vi "ASAP_SubVI_rt.vi"(6 "Reset":bool, 7 "Micron config":T1, 8 "error in":errorcluster, 9 "Configuration":T4, 10 "Time in":cluster{"t0":timestamp, "dt":dbl}, 11 "ADC data in":sgl[][](array[numeric])=[[0.4233891, 0.059737563, -0.3452632, -0.43708423, -0.1850327, 0.11627349, 0.3480983, 0.14520556, -0.018593404, -0.042756785, 0.0034736844, 0.02845318, -0.059975192, -0.3118025, -0.19130558, 0.09030185, 0.36043605], [0.6090162, 0.02373252, -0.52186435, -0.6243751, -0.2834785, 0.15024628, 0.48947865, 0.24355544, 0.052680574, 0.005137917, -0.03373152, -0.046069246, -0.18644089, -0.46828866, -0.19741842, 0.22753717, 0.5495514], [-0.36270568, 0.031333584, 0.3305598, 0.36922133, 0.17977042, -0.0914356, -0.29096755, -0.16731821, -0.07733762, -0.032019284, 0.04986418, 0.07868422, 0.16904892, 0.2834651, 0.064586245, -0.19497009, -0.3473115], [-0.6450181, 0.10571201, 0.61151254, 0.6368443, 0.17301747, -0.31877947, -0.51290303, -0.13209727, 0.06778669, 0.057593264, -0.031955272, -0.06567199, 0.19175611, 0.49285513, 0.23913881, -0.27019665, -0.6145497], [0.46957177, -0.13065708, -0.48157057, -0.46508822, -0.10884603, 0.27197546, 0.37166968, 0.08025244, -0.055926625, -0.03766807, 0.027317023, 0.049336106, -0.17896785, -0.37037078, -0.16486987, 0.23949087, 0.4787091], [0.6681609, -0.26571602, -0.7523299, -0.68411183, -0.18660091, 0.41935652, 0.55092764, 0.16146386, -0.011424401, -0.025378352, -0.01148841, -0.0049274913, -0.35867313, -0.5398829, -0.15688474, 0.44660845, 0.748461], [-0.3118825, 0.18517919, 0.40708274, 0.34915444, 0.12969938, -0.21727721, -0.29184768, -0.13747403, -0.0707447, -0.0026391712, 0.06805873, 0.0856772, 0.2530928, 0.25218067, -0.009680157, -0.29677638, -0.40475965], [-0.6122774, 0.44387203, 0.8820655, 0.6474379, 0.013395073, -0.6203265, -0.51136684, -0.011152362, 0.15547901, 0.035622187, -0.099948786, -0.11585501, 0.43435067, 0.58534867, 0.18177071, -0.5484282, -0.8615302], [-0.06624807, -0.05802292, -0.042420737, -0.031315185, -0.031459205, -0.04258076, -0.05151001, -0.051558014, -0.04872562, -0.048101533, -0.049829774, -0.051766045, -0.044020962, -0.033891544, -0.031091152, -0.04093253, -0.05603864], [-0.022401936, -0.022561958, -0.02249795, -0.022241915, -0.022017883, -0.022001881, -0.022113897, -0.022161903, -0.022225913, -0.022241915, -0.022321925, -0.022481948, -0.02243394, -0.022225913, -0.021953873, -0.021873862, -0.022113897], [-0.044613045, -0.04464505, -0.04464505, -0.04464505, -0.044629045, -0.044629045, -0.044629045, -0.044613045, -0.044613045, -0.044629045, -0.04459704, -0.044613045, -0.04464505, -0.044565037, -0.044613045, -0.044565037, -0.04458104], [-0.044565037, -0.044565037, -0.044533033, -0.044533033, -0.044549033, -0.044565037, -0.044549033, -0.04459704, -0.04451703, -0.044533033, -0.044533033, -0.044565037, -0.04459704, -0.044629045, -0.044613045, -0.044613045, -0.044613045]]) -> (0 "error out":errorcluster, 2 "Time out":cluster{"t0":timestamp, "dt":dbl}, 3 "XYZ out":sgl[][](array[numeric]) format="%#.2f", 4 "Position valid":bool, 5 "No pose":bool)   [LabVIEW 2014]
uses:
  initialization/configuration.ctl
  initialization/asap_calibration.ctl
  <vilib>/Analysis/Matrix/Datatypes/RealMatrix.ctl
  micron/labview/initialization/micron_config.ctl
  micron/labview/manipulator/squiggle/Host/i2c_interface.ctl
  micron/labview/manipulator/squiggle/Host/fpga_reference.ctl
  micron/labview/testing/Micron params.ctl
  micron/labview/testing/stimulus.ctl
  micron/labview/testing/injection_point.ctl
  micron/labview/filtering/goal_loop_parms.ctl
  micron/labview/testing/mode_conrols.ctl
  micron/labview/testing/manipulator_cal.ctl
  testing/probe_calibration.ctl
  micron/labview/host/network_params.ctl
  micron/labview/cancellation/sq_control_params.ctl
  micron/labview/cancellation/decoupled_gain.ctl
  micron/labview/cancellation/estimation_controls.ctl
  <vilib>/Analysis/4window.llb/Hanning Window (DBL).vi
  <vilib>/Analysis/4window.llb/AllCosWindow (DBL).vi
  <vilib>/Analysis/NI_AALPro.lvlib
  <vilib>/Analysis/Matrix/NI_Matrix.lvlib
panel:
  in  "Impulse filter":bool=TRUE
  in  "Window":bool=TRUE
  # "Options:"
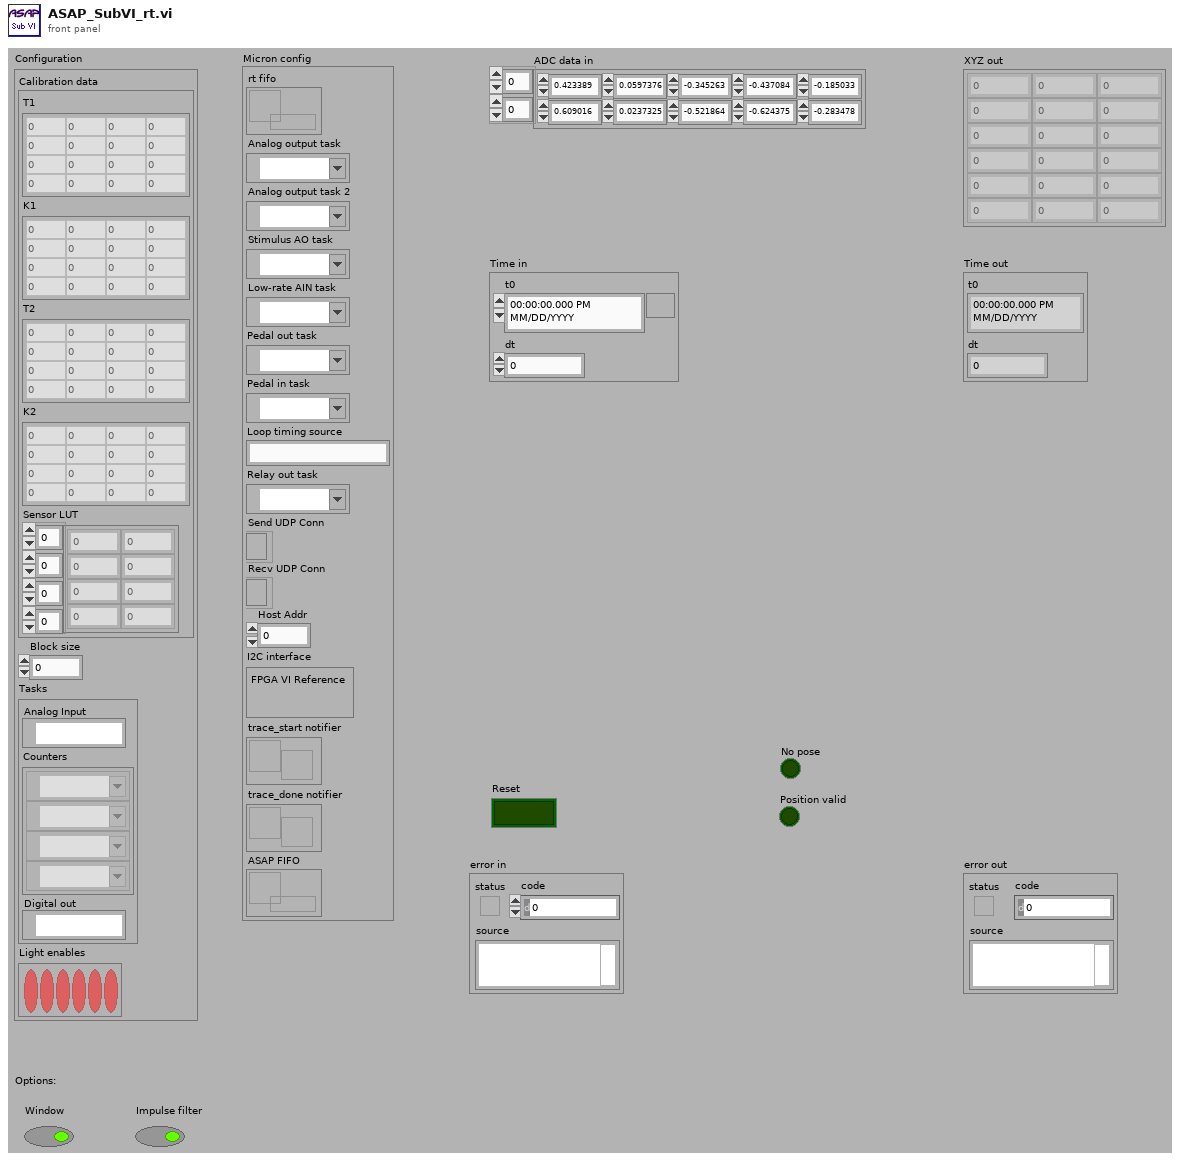
[diagram p1: front panel]
types:
  T1 = typedef "micron_config.ctl" = cluster{"rt fifo":refnum<k33>, "Analog output task":refnum<k21>, "Analog output task 2":refnum<k21>, "Stimulus AO task":refnum<k21>, "Low-rate AIN task":refnum<k21>, "Pedal out task":refnum<k21>, "Pedal in task":refnum<k21>, "Loop timing source":string, "Relay out task":refnum<k21>, "Send UDP Conn":refnum<k16>, "Recv UDP Conn":refnum<k16>, "Host Addr":u32, "I2C interface":T2, "trace_start notifier":refnum<notifier>, "trace_done notifier":refnum<notifier>, "ASAP FIFO":refnum<k33>}
  T2 = typedef "i2c_interface.ctl" = cluster{"FPGA VI Reference":T3}
  T3 = typedef "fpga_reference.ctl" = refnum<k20>
  T4 = typedef "configuration.ctl" = cluster{"Calibration data":T5, "Block size":i32, "Tasks":cluster{"Analog Input":refnum<k21>, "Counters":refnum<k21>[], "Digital out":refnum<k21>}, "Light enables":bool[]}
  T5 = typedef "asap_calibration.ctl" = cluster{"T1":T6, "K1":T6, "T2":T6, "K2":T6, "Sensor LUT":sgl[][][][]}
  T6 = typedef "NI_Matrix.lvlib/RealMatrix.ctl" = dbl[][]
  T7 = cluster{"Block size":i32, "Light enables":bool[], "Window":bool}
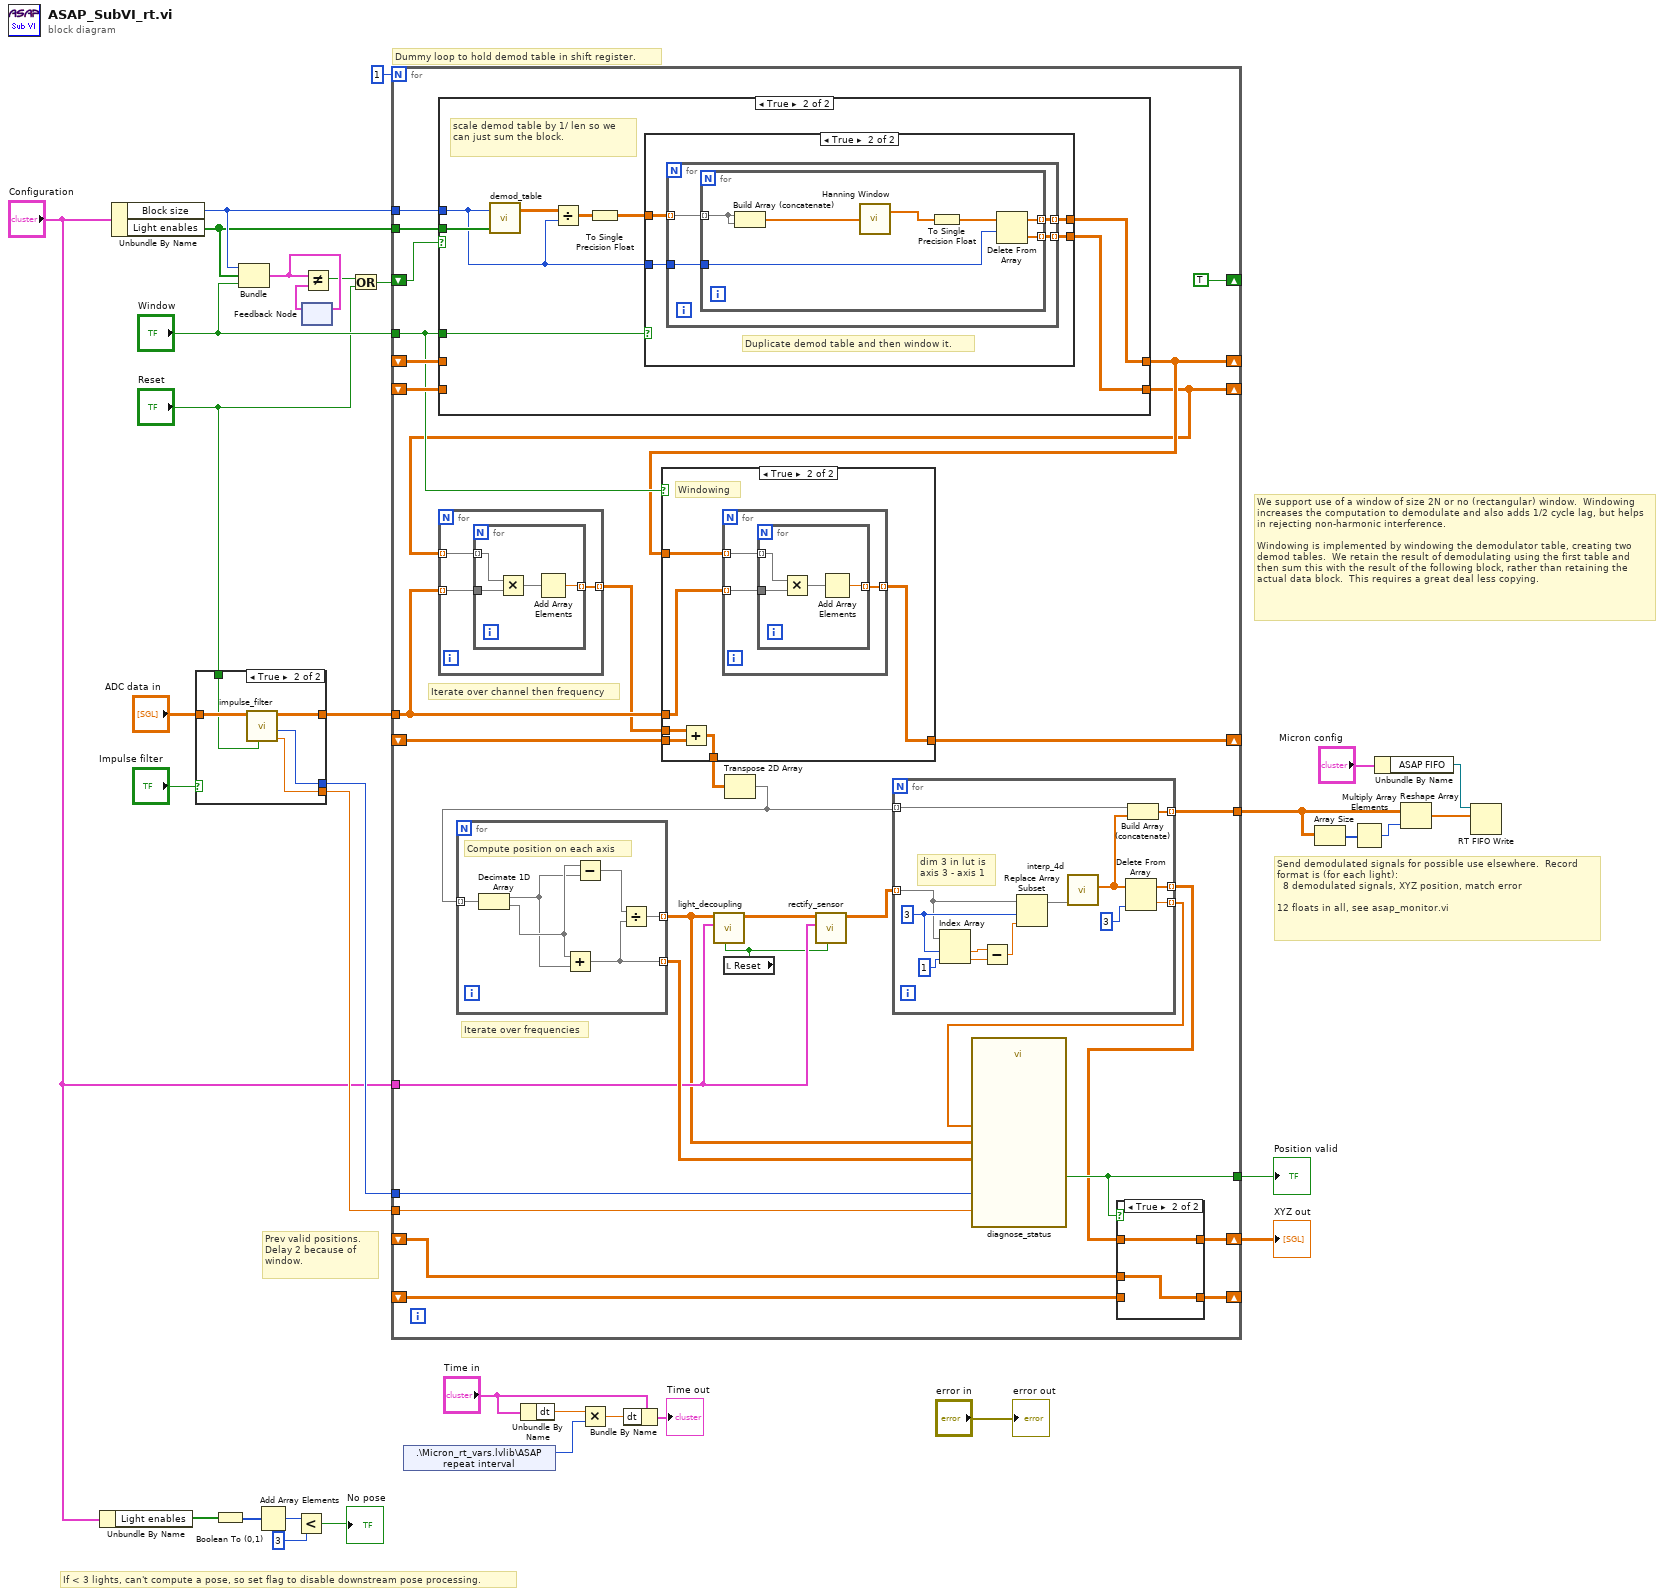
[diagram p0: block diagram]
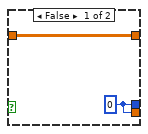
[diagram p2: hidden frame]
diagram:
  # "If < 3 lights, can't compute a pose, so set flag to disable downstream pose processing."
  # "Send demodulated signals for possible use elsewhere.  Record format is (for each light):\n  8 demodulated signals, XYZ position, match error\n\n12 floats in all, see asap_monitor.vi"
  # "Prev valid positions. Delay 2 because of window."
  # "We support use of a window of size 2N or no (rectangular) window.  Windowing increases the computation to demodulate and also adds 1/2 cycle lag, but helps in rejecting non-harmonic interference.\n\nWindowing is implemented by windowing the demodulator table, creating two demod tables.  We retain the result of demodulating using the first table and then sum this with the result of the following block, rather than retaining the actual data block.  This requires a great deal less copying."
  # "Dummy loop to hold demod table in shift register."
  n1 = Unbundle By Name("Configuration") -> ("Light enables"=w5:bool[])
  n2 = Unbundle By Name("Configuration") -> ("Block size"=w26:i32, "Light enables"=w25:bool[])
  n3 = case shown="True" "Impulse filter" {
    tunnel: "ADC data in" -> [w36 w39]
    tunnel: [w36 w38] -> w20
    tunnel: [w35 w41] -> w18
    tunnel: [w35 w40] -> w17
    tunnel: "Reset" -> [_ w37]
    frame False {
      w35 = 0 ("Repair count")
    }
    frame True {
      n4 = call "impulse_filter.vi"("Reset"=w37, "Signal in"=w39) -> ("RMS mismatch"=w40:sgl, "Repair count"=w41:i32, "Signal out"=w38:sgl[][])  [unwired: 7 in]
    }
  }
  n5 = Boolean To (0,1)(Boolean=w5) -> (0, 1=w4:i16[])
  n6 = Bundle("Block size"=w26, "Light enables"=w25, "Window"="Window") -> (w22:T7)  [unwired: 1 in]
  n7 = Add Array Elements(numeric array=w4) -> (sum=w3:i16)
  n8 = Less?(x=w3, y=i16 3) -> (x < y?=→"No pose":bool)
  n9 = feedback-in #1(w22) -> ()
  n10 = feedback #1() -> (w23:T7)  [unwired: 1 in]
  n11 = Not Equal?(x=w22, y=w23) -> (x != y?=w8:bool)
  n12 = Or(x=w8, y="Reset") -> (x .or. y?=w9:bool)
  n13 = for {
    N: 1 -> [_]
    tunnel: w20 -> [w64]
    shift-right: [w60] -> _
    shift-left: _ -> [w70]
    shift-right: [TRUE] -> _
    shift-left: w9 -> [w72]
    tunnel: w26 -> [w69]
    tunnel: w25 -> [w67]
    tunnel: [w51] -> w11
    shift-right: [w57] -> w28
    shift-left: _ -> [w56]
    tunnel: "Window" -> [w65]
    shift-right: [w59] -> _
    shift-left: _ -> [w66]
    shift-right: [w62] -> _
    shift-left: _ -> [w61]
    tunnel: [w46] -> w12
    shift-right: [w55] -> _
    shift-left: _ -> [w54]
    tunnel: w18 -> [w53]
    tunnel: w17 -> [w52]
    tunnel: "Configuration" -> [w45]
    # "Iterate over channel then frequency"
    # "Iterate over frequencies"
    n14 = case shown="True" w72 {
      tunnel: [w105 w107] -> w60
      tunnel: w70 -> [w105 _]
      tunnel: w69 -> [_ w108]
      tunnel: w67 -> [_ w111]
      tunnel: w65 -> [_ w110]
      tunnel: [w104 w106] -> w59
      tunnel: w66 -> [w104 _]
      frame False {
      }
      frame True {
        # "scale demod table by 1/ len so we can just sum the block."
        n15 = call "demod_table.vi"("Light enables"=w111, "Block size"=w108) -> ("Sine table"=w113:dbl[][][])  [unwired: 1 out]
        n16 = Divide(x=w113, y=w108) -> (x/y=w112:dbl[][][])
        n17 = To Single Precision Float(number=w112) -> (single precision float=w109:sgl[][][])
        n18 = case shown="True" w110 {
          tunnel: w109 -> [w114 w115]
          tunnel: w108 -> [_ w118]
          tunnel: [w114 w117] -> w107
          tunnel: [w114 w116] -> w106
          frame False {
          }
          frame True {
            # "Duplicate demod table and then window it."
            n19 = for {
              tunnel: w115 -> [w122] mode=indexing
              tunnel: [w121] -> w117 mode=indexing
              tunnel: [w120] -> w116 mode=indexing
              tunnel: w118 -> [w119]
              n20 = for {
                tunnel: w122 -> [w125] mode=indexing
                tunnel: [w129] -> w121 mode=indexing
                tunnel: [w128] -> w120 mode=indexing
                tunnel: w119 -> [w127]
                n21 = Build Array (concatenate)(w125, w125) -> (w123:sgl[])
                n22 = call-poly <vilib>:"Hanning Window.vi"("X"=w123) -> ("Windowed X"=w124:dbl[])  [unwired: 1 out]
                n23 = To Single Precision Float(number=w124) -> (single precision float=w126:sgl[])
                n24 = Delete From Array(array=w126, length=w127) -> (deleted portion=w128:sgl[], array with subset deleted=w129:sgl[])  [unwired: 1 in]
              }
            }
          }
        }
      }
    }
    n25 = for {
      tunnel: w64 -> [w132] mode=indexing
      tunnel: [w131] -> w63 mode=indexing
      tunnel: w59 -> [w130] mode=indexing
      n26 = for {
        tunnel: w132 -> [w136]
        tunnel: [w134] -> w131 mode=indexing
        tunnel: w130 -> [w133] mode=indexing
        n27 = Multiply(x=w133, y=w136) -> (x*y=w135:sgl[])
        n28 = Add Array Elements(numeric array=w135) -> (sum=w134:sgl)
      }
    }
    n29 = case shown="True" w65 {
      tunnel: w60 -> [_ w96]
      tunnel: w64 -> [_ w95]
      tunnel: w63 -> [w89 w94]
      tunnel: [w89 w93] -> w58
      tunnel: [w90 w92] -> w62
      tunnel: w61 -> [w90 w91]
      frame False {
        # "Not windowing"
      }
      frame True {
        # "Windowing"
        n30 = Add(x=w94, y=w91) -> (x+y=w93:sgl[][])
        n31 = for {
          tunnel: w95 -> [w99] mode=indexing
          tunnel: [w98] -> w92 mode=indexing
          tunnel: w96 -> [w97] mode=indexing
          n32 = for {
            tunnel: w99 -> [w103]
            tunnel: [w101] -> w98 mode=indexing
            tunnel: w97 -> [w100] mode=indexing
            n33 = Multiply(x=w100, y=w103) -> (x*y=w102:sgl[])
            n34 = Add Array Elements(numeric array=w102) -> (sum=w101:sgl)
          }
        }
      }
    }
    n35 = local read "Reset"() -> (w44:bool)
    n36 = Transpose 2D Array(2D array=w58) -> (transposed array=w47:sgl[][])
    n37 = for {
      tunnel: w47 -> [w142] mode=indexing
      tunnel: [w140] -> w68 mode=indexing
      tunnel: [w137] -> w42 mode=indexing
      # "Compute position on each axis"
      n38 = Decimate 1D Array(w142) -> (w139:sgl[], w141:sgl[])
      n39 = Add(x=w141, y=w139) -> (x+y=w140:sgl[])
      n40 = Subtract(x=w141, y=w139) -> (x-y=w138:sgl[])
      n41 = Divide(x=w138, y=w140) -> (x/y=w137:sgl[])
    }
    n42 = call "light_decoupling.vi"("Reset"=w44, "Configuration"=w45, "Array in"=w42) -> ("Array out"=w43:sgl[][])  [unwired: 8 in]
    n43 = call "rectify_sensor.vi"("Reset"=w44, "Configuration"=w45, "Array in"=w43) -> ("Array out"=w48:sgl[][])  [unwired: 8 in]
    n44 = for {
      tunnel: w48 -> [w78] mode=indexing
      tunnel: [w77] -> w49 mode=indexing
      tunnel: [w76] -> w50 mode=indexing
      tunnel: w47 -> [w75] mode=indexing
      tunnel: [w73] -> w46 mode=indexing
      w81 = 3 ("index (row)")
      # "dim 3 in lut is \naxis 3 - axis 1"
      n45 = Index Array(array=w78, index #1=w81, index #2=1 ("index (row)")) -> (element #1=w83:sgl, element #2=w84:sgl)
      n46 = Subtract(x=w83, y=w84) -> (x-y=w85:sgl)
      n47 = Replace Array Subset(array=w78, new element=w85, index=w81) -> (w80:sgl[])
      n48 = call "interp_4d.vi"("Input x"=w80) -> ("Output f(x)"=w74:sgl[])  [unwired: 2 in, 8 out]
      n49 = Delete From Array(array=w74, index=3) -> (deleted portion=w77:sgl, array with subset deleted=w76:sgl[])  [unwired: 1 in]
      n50 = Build Array (concatenate)(w75, w74) -> (w73:sgl[])
    }
    n51 = call "diagnose_status.vi"("RMS mismatch"=w52, "Repair count"=w53, "Axis positions"=w42, "Sum amplitudes"=w68, "Match error"=w49) -> ("Position valid"=w51:bool)  [unwired: 6 in]
    n52 = case shown="True" w51 {
      tunnel: [w86 w88] -> w57
      tunnel: w50 -> [_ w88]
      tunnel: w56 -> [_ w87]
      tunnel: [w86 w87] -> w55
      tunnel: w54 -> [w86 _]
      frame False {
      }
      frame True {
      }
    }
  }
  "XYZ out" <- w28
  "Position valid" <- w11
  n53 = shared-variable ".\\Micron_rt_vars.lvlib\\ASAP repeat interval"() -> (w27:i32)  [unwired: 2 out]
  n54 = Unbundle By Name("Time in") -> ("dt"=w33:dbl)
  n55 = Multiply(x=w33, y=w27) -> (x*y=w32:dbl)
  n56 = Bundle By Name(cluster="Time in", "dt"=w32) -> (→"Time out":cluster{"t0":timestamp, "dt":dbl})
  n57 = Array Size(array=w12) -> (size(s)=w14:i32[])
  n58 = Multiply Array Elements(1:w14) -> (0:w13:i32)
  n59 = Unbundle By Name("Micron config") -> ("ASAP FIFO"=w15:refnum<k33>)
  n60 = Reshape Array(w12, w13) -> (w10:sgl[])
  n61 = RT FIFO Write(0:w15, 1:w10) -> ()  [unwired: 2 in, 5 out]
  "error out" <- "error in"
